vi "SMTP Email Escape Header Word.vi"(1 "string":string) -> (0 "formated string":string)   [LabVIEW 2012, in "NewNI_SMTPEmail.lvlib"]
uses:
  NewNI_SMTPEmail.lvlib
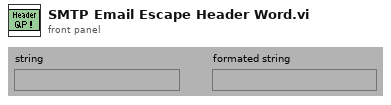
[diagram p1: front panel]
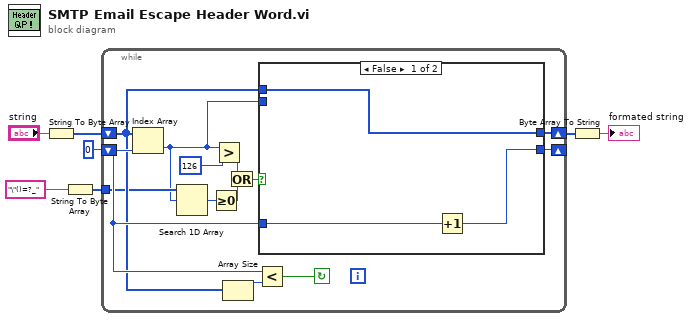
[diagram p0: block diagram]
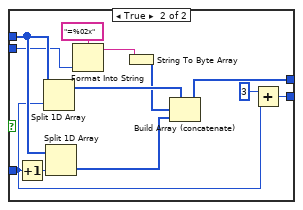
[diagram p2: hidden frame]
diagram:
  n1 = String To Byte Array(string="string") -> (unsigned byte array=w4:u8[])
  n2 = String To Byte Array(string="\"()=?_") -> (unsigned byte array=w5:u8[])
  n3 = while {
    tunnel: w5 -> [w9]
    shift-left: 0 -> [w15]
    shift-right: [w16] -> _
    shift-left: w4 -> [w14]
    shift-right: [w17] -> w3
    stop <- w19 continue-if-true
    n4 = Index Array(array=w14, index=w15) -> (element=w8:u8)
    n5 = Search 1D Array(1D array=w9, element=w8) -> (index of element=w10:i32)  [unwired: 1 out]
    n6 = Greater Or Equal To 0?(x=w10) -> (x >= 0?=w11:bool)
    n7 = Greater?(x=w8, y=u8 126) -> (0:w12:bool)
    n8 = Array Size(array=w14) -> (size(s)=w20:i32)
    n9 = Or(x=w12, y=w11) -> (x .or. y?=w13:bool)
    n10 = Less?(x=w15, y=w20) -> (x < y?=w19:bool)
    n11 = case shown="False" w13 {
      tunnel: w14 -> [w22 w35]
      tunnel: w15 -> [w23 w27]
      tunnel: w8 -> [_ w25]
      tunnel: [w22 w30] -> w17
      tunnel: [w21 w28] -> w16
      frame False {
        n12 = Increment(x=w23) -> (x+1=w21:i32)
      }
      frame True {
        n13 = Increment(x=w27) -> (x+1=w34:i32)
        n14 = Split 1D Array(array=w35, index=w27) -> (first subarray=w33:u8[])  [unwired: 1 out]
        n15 = Split 1D Array(array=w35, index=w34) -> (second subarray=w31:u8[])  [unwired: 1 out]
        n16 = Format Into String(format string="=%02x", w25) -> (resulting string=w24:string)  [unwired: 2 in, 1 out]
        n17 = String To Byte Array(string=w24) -> (unsigned byte array=w32:u8[])
        n18 = Build Array (concatenate)(w33, w32, w31) -> (w30:u8[])
        n19 = Add(x=3, y=w27) -> (x+y=w28:i32)
      }
    }
  }
  n20 = Byte Array To String(unsigned byte array=w3) -> (string=→"formated string":string)
